vi "Dashboard custom_bartender&global&gripper&camera2.vi"() -> ()   [LabVIEW 2017]
uses:
  C:/Users/IMR Lab/Documents/LabVIEW Data/UniversalRobotsSDK_LABView/LabVIEW/Examples/LabVIEW10/UnderAutomation.UniversalRobots.dll
  UnderAutomation.UniversalRobots.dll
  Global 1.vi
panel:
  out "Rz부호":string
  out "Ry부호":string
  out "Rx부호":string
  out "RZ_havetogo":string
  out "RY_havetogo":string
  out "RX_havetogo":string
  out "Z_havetogo":string
  out "Y_havetogo":string
  out "X_havetogo":string
  out "지호씨가보낸 총좌표":string
  out "TCPOffsetRZ":dbl
  out "TCPOffsetRY":dbl
  out "TCPOffsetRX":dbl
  out "TCPOffsetZ":dbl
  out "TCPOffsetY":dbl
  out "TCPOffsetX":dbl
  out "3rd Order":bool
  out "2nd Order":bool
  out "1st Order":bool
  in  "stop":bool
  out "Rx":dbl
  out "Rz":dbl
  out "Ry":dbl
  out "Enabled":bool
  out "Port":i32
  in  "Move to particular posture":bool
  in  "Move to Zero position":bool
  out "Connected":bool
  in  "Robot IP(192.168.112.182)":string
  out "Connect error":errorcluster
  in  "Power on\nRelease brake":bool
  in  "Power off":bool
  in  "Connect":bool
  in  "Send script":bool
  in  "Script to execute":string
  out "Powered on":bool
  out "X":dbl
  out "Y":dbl
  out "Z":dbl
  out "License state":string
  # "랩뷰가 보여주는 RX RY RZ 는 신뢰x"
  # "movel(p[-0.0753945, -0.304532, 0.314608, -0.194623, 2.71667, -1.00228], a= 0.5, v=0.25)"
  # "movej( get_inverse_kin(p[0.3138, 0.0814, 0.1647, 0.4226, -2.3876, -2.3851]),  a=0.5, v=0.25, t=0, r=0)"
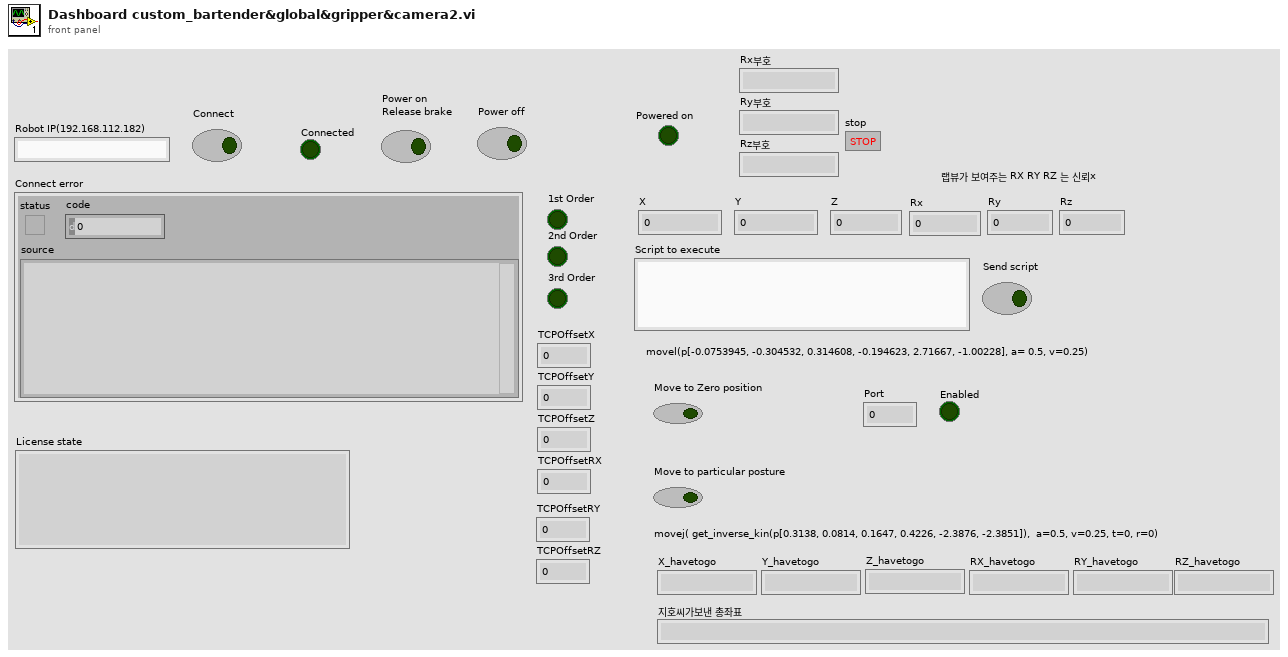
[diagram p1: front panel]
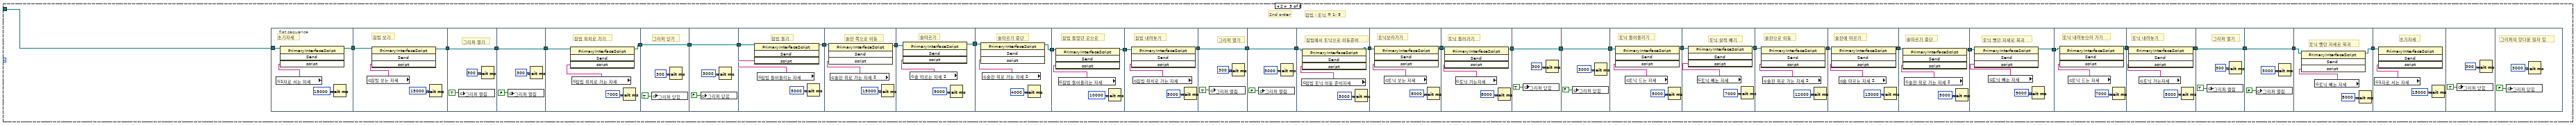
[diagram p14: hidden frame]
diagram:
  # "미니콜라 따르는 자세"
  # "술잔 중간지점 가는 자세"
  # "짐빔에서 토닉이동 준비 자세"
  # "술잔 따르는 자세2"
  # "술잔 위로 가는 자세2"
  # "토닉워터 뺴는 자세"
  # "토닉워 들어올리는 자세"
  # "토닉워터 가는 자세"
  # "토닉워터 보는 자세"
  # "짐빔 들어올리는 자세"
  # "짐빔로 가는 자세"
  # "짐빔 보는 자세"
  # "콜라 뺴는 자세"
  # "콜라 들어올리는 자세"
  # "콜라로 가는 자세"
  # "콜라 보는 자세"
  # "술잔 따르는 자세"
  # "술잔 위로 가는 자세"
  # "잭다니엘 들어올리는 자세"
  # "잭다니엘 위치로 가는 자세"
  # "잭다니엘 보는 자세"
  # "1자로 서는 자세"
  # "Example : Display power on status"
  # "Create a UR\ncobot instance"
  # "Show license state"
  # "Register your confidential license key to exit\ntrial period and use this library forever"
  # "Power off when button is clicked"
  # "Power on and release brake when button is clicked"
  # "Get your UR Dashboard interface"
  n1 = global write "Global 1.vi" "미니콜라 따르는 자세"("movej([-0.0902,-1.8120,-1.9241,-3.5769,6.2827,8.4658], a=0.5, v=0.25, t=0, r=0)") -> ()
  n2 = global write "Global 1.vi" "술잔 중간지점"("movej([-0.2173,-1.9485,-1.6874,-3.9352,6.2671,7.2276], a=0.5, v=0.25, t=0, r=0)") -> ()
  n3 = global write "Global 1.vi" "짐빔 토닉 이동 준비자세"("movej([-0.5421,-0.8131,0.8439,-0.0538,2.5052,5.9032], a=0.5, v=0.25, t=0, r=0)") -> ()
  n4 = global write "Global 1.vi" "잭다니엘 들어올리는 자세"("movej([0.8116,-2.0223,-1.2828,-3.0107,4.3284,5.9341], a=0.5, v=0.25, t=0, r=0)") -> ()
  n5 = global write "Global 1.vi" "잭다닐 위치로 가는 자세"("movej([0.8116,-2.3119,-1.606,-2.3958,4.3284,5.9341], a=0.5, v=0.25, t=0, r=0)") -> ()
  n6 = global write "Global 1.vi" "짐빔 들어올리는 자세"("movej([-0.5421,-0.8131,0.8439,-0.0538,2.5052,5.9032], a=0.5, v=0.25, t=0, r=0)") -> ()
  n7 = global write "Global 1.vi" "술잔 위로 가는 자세 2"("movej([0.0485,-1.6015,2.5780,-1.0382,-0.0520,5.3649], a=0.5, v=0.25, t=0, r=0)") -> ()
  n8 = global write "Global 1.vi" "1자로 서는 자세"("movej([3.1412,-1.5708,0,-1.5708,3.1412,5.8904], a=0.5, v=0.25, t=0, r=0)") -> ()
  n9 = global write "Global 1.vi" "짐빔 위치로 가는 자세"("movej([-0.5436,-0.4519,0.8428,-0.3534,2.6134,5.9032], a=0.5, v=0.25, t=0, r=0)") -> ()
  n10 = global write "Global 1.vi" "술잔 위로 가는 자세"("movej([-0.0903,-2.0548,-2.0169,-3.3289,6.2826,7.4091], a=0.5, v=0.25, t=0, r=0)") -> ()
  n11 = global write "Global 1.vi" "잭다니엘 보는 자세"("movej([0,-2.2170,-1.4226,-2.2842,3.1412,6.2832], a=0.5, v=0.25, t=0, r=0)") -> ()
  n12 = global write "Global 1.vi" "콜라 빼는 자세"("movej([0.8789,-1.5237,-2.1070,-2.6679, 3.9917,5.9085], a=0.5, v=0.25, t=0, r=0)") -> ()
  n13 = global write "Global 1.vi" "콜라 드는 자세"("movej([1.2020,-1.8452,-1.7403,-2.7082,4.3162,5.9158], a=0.5, v=0.25, t=0, r=0)") -> ()
  n14 = global write "Global 1.vi" "콜라 보는 자세"("movej([0,-1.8110,-2.1684,-2.3033,3.1543,5.9213], a=0.5, v=0.25, t=0, r=0)") -> ()
  n15 = global write "Global 1.vi" "콜라로 가는자세"("movej([1.2020,-2.166,-1.9385,-2.1863,4.3172,5.9210], a=0.5, v=0.25, t=0, r=0)") -> ()
  n16 = global write "Global 1.vi" "토닉 빼는 자세"("movej([-0.5277,-1.5104,1.5889,-0.0548,2.5728,5.9025], a=0.5, v=0.25, t=0, r=0)") -> ()
  n17 = global write "Global 1.vi" "술 따르는 자세 2"("movej([0.0412,-1.9708,2.4700,-1.0157,-0.0618,4.8998], a=0.5, v=0.25, t=0, r=0)") -> ()
  n18 = global write "Global 1.vi" "짐빔 보는 자세"("movej([-0.0364,-0.6154,0.9421,-0.3291,3.1047,5.9020], a=0.5, v=0.25, t=0, r=0)") -> ()
  n19 = global write "Global 1.vi" "토닉 드는 자세"("movej([-1.0311,-1.1460,1.5830,-0.4348,2.0708,5.9048], a=0.5, v=0.25, t=0, r=0)") -> ()
  n20 = global write "Global 1.vi" "토닉 보는 자세"("movej([-0.4690,-1.1292,2.1508,-1.0119,2.6124,5.9032], a=0.5, v=0.25, t=0, r=0)") -> ()
  n21 = global write "Global 1.vi" "술 따르는 자세"("movej([-0.0902,-1.9024,-1.9241,-3.5769,6.2827,8.4692], a=0.5, v=0.25, t=0, r=0)") -> ()
  n22 = global write "Global 1.vi" "토닉 가는자세"("movej([-0.9924,-0.8742,1.7459,-0.8837,2.0958,5.9048], a=0.5, v=0.25, t=0, r=0)") -> ()
  n23 = constructor class="UR"() -> (reference out=w25:refnum<k24>)  [unwired: 3 in, 2 out]
  n24 = while {
    tunnel: w25 -> [w31]
    stop <- FALSE stop-if-true
    # "Connect to the robot when button is pressed"
    # "Show if primary interface is connected"
    # "Get your UR primary interface"
    n25 = property class="UR"(reference=w31) -> ("PrimaryInterface"=w34:refnum<k24>)  [unwired: 1 in, 2 out]
    n26 = Wait (ms)(milliseconds to wait=u32 50) -> ()  [unwired: 1 out]
    n27 = property class="PrimaryInterfaceClientInternal"(reference=w34) -> ("Connected"=w33:bool)  [unwired: 1 in, 2 out]
    "Connected" <- w33
    n28 = case shown="True" "Connect" {
      tunnel: w31 -> [_ w478]
      frame False {
      }
      frame True {
        n29 = flat-sequence {
          tunnel: w478 -> [w480]
          frame #0 {
            n30 = invoke class="UR" method="Connect"(reference=w480, "ip"="Robot IP(192.168.112.182)") -> (error out=→"Connect error":errorcluster)  [unwired: 2 in, 3 out]
          }
        }
      }
    }
    n31 = case shown="True" w33 {
      tunnel: w34 -> [_ w40]
      frame False {
      }
      frame True {
        # "Send URScript when button pressed"
        # "Example : Display current cartesian pose"
        n32 = property class="PrimaryInterfaceClientInternal"(reference=w40) -> ("Script"=w48:refnum<k24>)  [unwired: 1 in, 2 out]
        n33 = global read "Global 1.vi" "2nd Order"() -> (w51:bool)
        "2nd Order" <- w51
        n34 = global read "Global 1.vi" "3rd Order"() -> (w50:bool)
        "3rd Order" <- w50
        n35 = global read "Global 1.vi" "1st Order"() -> (w52:bool)
        "1st Order" <- w52
        n36 = Build Array(w52, w51, w50) -> (w53:bool[])
        n37 = Boolean Array To Number(Boolean array=w53) -> (number=w49:u32)
        n38 = case shown="1" w49 {
          tunnel: w48 -> [_ w106 w313 _ _ _ _ _]
          frame 0, Default {
          }
          frame 1 {
            # "잭다 : 콜라 = 1 : 3"
            # "1st order"
            n39 = flat-sequence {
              tunnel: w106 -> [w110]
              tunnel: [w109] -> w105
              tunnel: w105 -> [w114]
              tunnel: [w112] -> w97
              tunnel: w97 -> [w117]
              tunnel: [w117] -> w95
              tunnel: w95 -> [w120]
              tunnel: [w120] -> w72
              tunnel: w72 -> [w124]
              tunnel: [w124] -> w69
              tunnel: w69 -> [w128]
              tunnel: [w128] -> w68
              tunnel: w68 -> [w190]
              tunnel: [w190] -> w71
              tunnel: w71 -> [w191]
              tunnel: [w191] -> w70
              tunnel: w70 -> [w195]
              tunnel: [w192] -> w96
              tunnel: w96 -> [w198]
              tunnel: [w198] -> w94
              tunnel: w94 -> [w201]
              tunnel: [w201] -> w93
              tunnel: w93 -> [w203]
              tunnel: [w202] -> w80
              tunnel: w80 -> [w207]
              tunnel: [w206] -> w79
              tunnel: w79 -> [w211]
              tunnel: [w210] -> w104
              tunnel: w104 -> [w216]
              tunnel: [w214] -> w103
              tunnel: w103 -> [w219]
              tunnel: [w218] -> w78
              tunnel: w78 -> [w223]
              tunnel: [w222] -> w77
              tunnel: [w226] -> w102
              tunnel: w77 -> [w228]
              tunnel: w102 -> [w231]
              tunnel: [w230] -> w92
              tunnel: w92 -> [w236]
              tunnel: [w236] -> w91
              tunnel: w91 -> [w239]
              tunnel: [w239] -> w90
              tunnel: w90 -> [w241]
              tunnel: [w240] -> w101
              tunnel: w101 -> [w245]
              tunnel: [w244] -> w89
              tunnel: w89 -> [w250]
              tunnel: [w250] -> w88
              tunnel: w88 -> [w253]
              tunnel: [w253] -> w87
              tunnel: w87 -> [w255]
              tunnel: [w254] -> w86
              tunnel: w86 -> [w259]
              tunnel: [w258] -> w76
              tunnel: w76 -> [w263]
              tunnel: [w262] -> w75
              tunnel: w75 -> [w267]
              tunnel: [w266] -> w100
              tunnel: w100 -> [w271]
              tunnel: [w270] -> w99
              tunnel: w99 -> [w275]
              tunnel: [w274] -> w74
              tunnel: w74 -> [w279]
              tunnel: [w278] -> w73
              tunnel: w73 -> [w283]
              tunnel: [w282] -> w85
              tunnel: w85 -> [w287]
              tunnel: [w286] -> w98
              tunnel: w98 -> [w291]
              tunnel: [w290] -> w83
              tunnel: [w294] -> w84
              tunnel: w83 -> [w294]
              tunnel: [w297] -> w82
              tunnel: w84 -> [w297]
              tunnel: w82 -> [w301]
              tunnel: [w300] -> w81
              tunnel: w81 -> [w304]
              frame #0 {
                # "초기자세"
                n40 = global read "Global 1.vi" "1자로 서는 자세"() -> (w108:string)
                n41 = invoke class="PrimaryInterfaceScript" method="Send"(reference=w110, "script"=w108) -> (reference out=w109:refnum<k24>)  [unwired: 2 in, 3 out]
                n42 = Wait (ms)(milliseconds to wait=u32 15000) -> ()  [unwired: 1 out]
              }
              frame #1 {
                # "잭다니엘 보기"
                n43 = global read "Global 1.vi" "잭다니엘 보는 자세"() -> (w113:string)
                n44 = invoke class="PrimaryInterfaceScript" method="Send"(reference=w114, "script"=w113) -> (reference out=w112:refnum<k24>)  [unwired: 2 in, 3 out]
                n45 = Wait (ms)(milliseconds to wait=u32 15000) -> ()  [unwired: 1 out]
              }
              frame #2 {
                # "그리퍼 열기"
                n46 = global write "Global 1.vi" "그리퍼 열림"(TRUE ("그리퍼 열림")) -> ()
                n47 = Wait (ms)(milliseconds to wait=u32 300) -> ()  [unwired: 1 out]
              }
              frame #3 {
                n48 = global write "Global 1.vi" "그리퍼 열림"(FALSE ("그리퍼 열림")) -> ()
                n49 = Wait (ms)(milliseconds to wait=u32 300) -> ()  [unwired: 1 out]
              }
              frame #4 {
                n50 = global write "Global 1.vi" "몇번 병을 볼것인가"("0" ("몇번 병을 볼것인가")) -> ()
                n51 = global write "Global 1.vi" "TCP 스위치"(TRUE ("그리퍼 열림")) -> ()
                n52 = Wait (ms)(milliseconds to wait=u32 300) -> ()  [unwired: 1 out]
              }
              frame #5 {
                n53 = local read "Rx부호"() -> (w127:string)
                n54 = local read "Ry부호"() -> (w126:string)
                n55 = local read "Rz부호"() -> (w125:string)
                n56 = case shown="\"1\"" w125 {
                  frame "False", Default {
                  }
                  frame "True" {
                  }
                  frame "2" {
                  }
                  frame "1" {
                    n57 = local read "RZ_havetogo"() -> (w133:string)
                    n58 = Decimal String To Number(string=w133) -> (number=w132:i32)  [unwired: 2 in, 1 out]
                    n59 = To Double Precision Float(number=w132) -> (double precision float=w131:dbl)
                    n60 = Format Into String(format string="-%f", w131) -> (resulting string=w129:string)  [unwired: 2 in, 1 out]
                    n61 = local write "RZ_havetogo"(w129) -> ()
                  }
                }
                n62 = case shown="\"1\"" w126 {
                  frame "False", Default {
                  }
                  frame "True" {
                  }
                  frame "2" {
                  }
                  frame "1" {
                    n63 = local read "RY_havetogo"() -> (w138:string)
                    n64 = Decimal String To Number(string=w138) -> (number=w137:i32)  [unwired: 2 in, 1 out]
                    n65 = To Double Precision Float(number=w137) -> (double precision float=w134:dbl)
                    n66 = Format Into String(format string="-%f", w134) -> (resulting string=w135:string)  [unwired: 2 in, 1 out]
                    n67 = local write "RY_havetogo"(w135) -> ()
                  }
                }
                n68 = case shown="\"1\"" w127 {
                  frame "False", Default {
                  }
                  frame "True" {
                  }
                  frame "2" {
                  }
                  frame "1" {
                    n69 = local read "RX_havetogo"() -> (w143:string)
                    n70 = Decimal String To Number(string=w143) -> (number=w142:i32)  [unwired: 2 in, 1 out]
                    n71 = To Double Precision Float(number=w142) -> (double precision float=w141:dbl)
                    n72 = Format Into String(format string="-%f", w141) -> (resulting string=w139:string)  [unwired: 2 in, 1 out]
                    n73 = local write "RX_havetogo"(w139) -> ()
                  }
                }
              }
              frame #6 {
                n74 = local read "RZ_havetogo"() -> (w182:string)
                n75 = local read "RY_havetogo"() -> (w183:string)
                n76 = local read "Y_havetogo"() -> (w186:string)
                n77 = local read "Z_havetogo"() -> (w185:string)
                n78 = local read "RX_havetogo"() -> (w184:string)
                n79 = local read "X_havetogo"() -> (w187:string)
                n80 = Decimal String To Number(string=w185) -> (number=w173:i32)  [unwired: 2 in, 1 out]
                n81 = Decimal String To Number(string=w187) -> (number=w179:i32)  [unwired: 2 in, 1 out]
                n82 = Decimal String To Number(string=w186) -> (number=w176:i32)  [unwired: 2 in, 1 out]
                n83 = Decimal String To Number(string=w184) -> (number=w170:i32)  [unwired: 2 in, 1 out]
                n84 = Decimal String To Number(string=w183) -> (number=w167:i32)  [unwired: 2 in, 1 out]
                n85 = Decimal String To Number(string=w182) -> (number=w164:i32)  [unwired: 2 in, 1 out]
                n86 = To Double Precision Float(number=w179) -> (double precision float=w181:dbl)
                n87 = To Double Precision Float(number=w173) -> (double precision float=w175:dbl)
                n88 = To Double Precision Float(number=w176) -> (double precision float=w178:dbl)
                n89 = To Double Precision Float(number=w170) -> (double precision float=w172:dbl)
                n90 = To Double Precision Float(number=w167) -> (double precision float=w169:dbl)
                n91 = local read "X"() -> (w151:dbl)
                n92 = Multiply(x=w181, y=0.001) -> (x*y=w163:dbl)
                n93 = Multiply(x=w175, y=0.001) -> (x*y=w159:dbl)
                n94 = Multiply(x=w178, y=0.001) -> (x*y=w161:dbl)
                n95 = Multiply(x=w172, y=0.001) -> (x*y=w157:dbl)
                n96 = Multiply(x=w169, y=0.001) -> (x*y=w155:dbl)
                n97 = local read "Y"() -> (w150:dbl)
                n98 = local read "Z"() -> (w149:dbl)
                n99 = To Double Precision Float(number=w164) -> (double precision float=w166:dbl)
                n100 = Add(x=w151, y=w163) -> (x+y=w162:dbl)
                n101 = local read "Rx"() -> (w148:dbl)
                n102 = Multiply(x=w166, y=0.001) -> (x*y=w153:dbl)
                n103 = Add(x=w159, y=w149) -> (x+y=w158:dbl)
                n104 = Add(x=w161, y=w150) -> (x+y=w160:dbl)
                n105 = local read "Ry"() -> (w147:dbl)
                n106 = local read "Rz"() -> (w146:dbl)
                n107 = Add(x=w157, y=w148) -> (x+y=w156:dbl)
                n108 = Add(x=w155, y=w147) -> (x+y=w154:dbl)
                n109 = Add(x=w153, y=w146) -> (x+y=w152:dbl)
                n110 = Format Into String(format string="movej( get_inverse_kin(p[%f, %f, %f, %f, %f, %f]), a= 0.5, v=0.25, t=0, r=0)", w162, w160, w158, w156, w154, w152) -> (resulting string=w144:string)  [unwired: 2 in, 1 out]
                n111 = global write "Global 1.vi" "잭다닐 위치로 가는 자세"(w144) -> ()
                n112 = global write "Global 1.vi" "TCP 스위치"(FALSE ("그리퍼 열림")) -> ()
                n113 = Wait (ms)(milliseconds to wait=u32 300) -> ()  [unwired: 1 out]
              }
              frame #7 {
              }
              frame #8 {
                # "잭다니엘 위치로 가기"
                n114 = global read "Global 1.vi" "잭다닐 위치로 가는 자세"() -> (w194:string)
                n115 = invoke class="PrimaryInterfaceScript" method="Send"(reference=w195, "script"=w194) -> (reference out=w192:refnum<k24>)  [unwired: 2 in, 3 out]
                n116 = Wait (ms)(milliseconds to wait=u32 7000) -> ()  [unwired: 1 out]
              }
              frame #9 {
                # "그리퍼 닫기"
                n117 = global write "Global 1.vi" "그리퍼 닫힘"(TRUE ("그리퍼 열림")) -> ()
                n118 = Wait (ms)(milliseconds to wait=u32 300) -> ()  [unwired: 1 out]
              }
              frame #10 {
                n119 = global write "Global 1.vi" "그리퍼 닫힘"(FALSE ("그리퍼 열림")) -> ()
                n120 = Wait (ms)(milliseconds to wait=u32 3000) -> ()  [unwired: 1 out]
              }
              frame #11 {
                # "잭다니엘 들기"
                n121 = global read "Global 1.vi" "잭다니엘 들어올리는 자세"() -> (w205:string)
                n122 = invoke class="PrimaryInterfaceScript" method="Send"(reference=w203, "script"=w205) -> (reference out=w202:refnum<k24>)  [unwired: 2 in, 3 out]
                n123 = Wait (ms)(milliseconds to wait=u32 3000) -> ()  [unwired: 1 out]
              }
              frame #12 {
                # "술잔 중간지점으로 이동"
                n124 = global read "Global 1.vi" "술잔 중간지점"() -> (w208:string)
                n125 = invoke class="PrimaryInterfaceScript" method="Send"(reference=w207, "script"=w208) -> (reference out=w206:refnum<k24>)  [unwired: 2 in, 3 out]
                n126 = Wait (ms)(milliseconds to wait=u32 15000) -> ()  [unwired: 1 out]
              }
              frame #13 {
                # "술잔 쪽으로 이동"
                n127 = global read "Global 1.vi" "술잔 위로 가는 자세"() -> (w212:string)
                n128 = invoke class="PrimaryInterfaceScript" method="Send"(reference=w211, "script"=w212) -> (reference out=w210:refnum<k24>)  [unwired: 2 in, 3 out]
                n129 = Wait (ms)(milliseconds to wait=u32 5000) -> ()  [unwired: 1 out]
              }
              frame #14 {
                # "술따르기"
                n130 = global read "Global 1.vi" "술 따르는 자세"() -> (w215:string)
                n131 = invoke class="PrimaryInterfaceScript" method="Send"(reference=w216, "script"=w215) -> (reference out=w214:refnum<k24>)  [unwired: 2 in, 3 out]
                n132 = Wait (ms)(milliseconds to wait=u32 9000) -> ()  [unwired: 1 out]
              }
              frame #15 {
                # "술따르기 중단"
                n133 = global read "Global 1.vi" "술잔 위로 가는 자세"() -> (w220:string)
                n134 = invoke class="PrimaryInterfaceScript" method="Send"(reference=w219, "script"=w220) -> (reference out=w218:refnum<k24>)  [unwired: 2 in, 3 out]
                n135 = Wait (ms)(milliseconds to wait=u32 4000) -> ()  [unwired: 1 out]
              }
              frame #16 {
                # "술잔 중간지점으로 이동"
                n136 = global read "Global 1.vi" "술잔 중간지점"() -> (w224:string)
                n137 = invoke class="PrimaryInterfaceScript" method="Send"(reference=w223, "script"=w224) -> (reference out=w222:refnum<k24>)  [unwired: 2 in, 3 out]
                n138 = Wait (ms)(milliseconds to wait=u32 7000) -> ()  [unwired: 1 out]
              }
              frame #17 {
                # "잭다니엘 들었던 곳으로"
                n139 = global read "Global 1.vi" "잭다니엘 들어올리는 자세"() -> (w227:string)
                n140 = invoke class="PrimaryInterfaceScript" method="Send"(reference=w228, "script"=w227) -> (reference out=w226:refnum<k24>)  [unwired: 2 in, 3 out]
                n141 = Wait (ms)(milliseconds to wait=u32 10000) -> ()  [unwired: 1 out]
              }
              frame #18 {
                # "잭다니엘 내려놓기"
                n142 = global read "Global 1.vi" "잭다닐 위치로 가는 자세"() -> (w233:string)
                n143 = invoke class="PrimaryInterfaceScript" method="Send"(reference=w231, "script"=w233) -> (reference out=w230:refnum<k24>)  [unwired: 2 in, 3 out]
                n144 = Wait (ms)(milliseconds to wait=u32 5000) -> ()  [unwired: 1 out]
              }
              frame #19 {
                # "그리퍼 열기"
                n145 = global write "Global 1.vi" "그리퍼 열림"(TRUE ("그리퍼 열림")) -> ()
                n146 = Wait (ms)(milliseconds to wait=u32 300) -> ()  [unwired: 1 out]
              }
              frame #20 {
                n147 = global write "Global 1.vi" "그리퍼 열림"(FALSE ("그리퍼 열림")) -> ()
                n148 = Wait (ms)(milliseconds to wait=u32 3000) -> ()  [unwired: 1 out]
              }
              frame #21 {
                # "콜라보러가기"
                n149 = global read "Global 1.vi" "콜라 보는 자세"() -> (w243:string)
                n150 = invoke class="PrimaryInterfaceScript" method="Send"(reference=w241, "script"=w243) -> (reference out=w240:refnum<k24>)  [unwired: 2 in, 3 out]
                n151 = Wait (ms)(milliseconds to wait=u32 8000) -> ()  [unwired: 1 out]
              }
              frame #22 {
                # "콜라 들러가기"
                n152 = global read "Global 1.vi" "콜라로 가는자세"() -> (w247:string)
                n153 = invoke class="PrimaryInterfaceScript" method="Send"(reference=w245, "script"=w247) -> (reference out=w244:refnum<k24>)  [unwired: 2 in, 3 out]
                n154 = Wait (ms)(milliseconds to wait=u32 8000) -> ()  [unwired: 1 out]
              }
              frame #23 {
                n155 = global write "Global 1.vi" "그리퍼 닫힘"(TRUE ("그리퍼 열림")) -> ()
                n156 = Wait (ms)(milliseconds to wait=u32 300) -> ()  [unwired: 1 out]
              }
              frame #24 {
                n157 = global write "Global 1.vi" "그리퍼 닫힘"(FALSE ("그리퍼 열림")) -> ()
                n158 = Wait (ms)(milliseconds to wait=u32 3000) -> ()  [unwired: 1 out]
              }
              frame #25 {
                # "콜라 들어올리기"
                n159 = global read "Global 1.vi" "콜라 드는 자세"() -> (w257:string)
                n160 = invoke class="PrimaryInterfaceScript" method="Send"(reference=w255, "script"=w257) -> (reference out=w254:refnum<k24>)  [unwired: 2 in, 3 out]
                n161 = Wait (ms)(milliseconds to wait=u32 5000) -> ()  [unwired: 1 out]
              }
              frame #26 {
                # "콜라 살짝 빼기"
                n162 = global read "Global 1.vi" "콜라 빼는 자세"() -> (w261:string)
                n163 = invoke class="PrimaryInterfaceScript" method="Send"(reference=w259, "script"=w261) -> (reference out=w258:refnum<k24>)  [unwired: 2 in, 3 out]
                n164 = Wait (ms)(milliseconds to wait=u32 5000) -> ()  [unwired: 1 out]
              }
              frame #27 {
                # "술잔 중간지점으로 이동"
                n165 = global read "Global 1.vi" "술잔 중간지점"() -> (w264:string)
                n166 = invoke class="PrimaryInterfaceScript" method="Send"(reference=w263, "script"=w264) -> (reference out=w262:refnum<k24>)  [unwired: 2 in, 3 out]
                n167 = Wait (ms)(milliseconds to wait=u32 15000) -> ()  [unwired: 1 out]
              }
              frame #28 {
                # "술잔으로 이동"
                n168 = global read "Global 1.vi" "술잔 위로 가는 자세"() -> (w269:string)
                n169 = invoke class="PrimaryInterfaceScript" method="Send"(reference=w267, "script"=w269) -> (reference out=w266:refnum<k24>)  [unwired: 2 in, 3 out]
                n170 = Wait (ms)(milliseconds to wait=u32 5000) -> ()  [unwired: 1 out]
              }
              frame #29 {
                # "미니콜라에 따르기"
                n171 = global read "Global 1.vi" "미니콜라 따르는 자세"() -> (w273:string)
                n172 = invoke class="PrimaryInterfaceScript" method="Send"(reference=w271, "script"=w273) -> (reference out=w270:refnum<k24>)  [unwired: 2 in, 3 out]
                n173 = Wait (ms)(milliseconds to wait=u32 11000) -> ()  [unwired: 1 out]
              }
              frame #30 {
                # "술따르기 중단"
                n174 = global read "Global 1.vi" "술잔 위로 가는 자세"() -> (w277:string)
                n175 = invoke class="PrimaryInterfaceScript" method="Send"(reference=w275, "script"=w277) -> (reference out=w274:refnum<k24>)  [unwired: 2 in, 3 out]
                n176 = Wait (ms)(milliseconds to wait=u32 5000) -> ()  [unwired: 1 out]
              }
              frame #31 {
                # "술잔 중간지점으로 이동"
                n177 = global read "Global 1.vi" "술잔 중간지점"() -> (w280:string)
                n178 = invoke class="PrimaryInterfaceScript" method="Send"(reference=w279, "script"=w280) -> (reference out=w278:refnum<k24>)  [unwired: 2 in, 3 out]
                n179 = Wait (ms)(milliseconds to wait=u32 7000) -> ()  [unwired: 1 out]
              }
              frame #32 {
                # "콜라 뻇던 자세로 복귀"
                n180 = global read "Global 1.vi" "콜라 빼는 자세"() -> (w284:string)
                n181 = invoke class="PrimaryInterfaceScript" method="Send"(reference=w283, "script"=w284) -> (reference out=w282:refnum<k24>)  [unwired: 2 in, 3 out]
                n182 = Wait (ms)(milliseconds to wait=u32 7000) -> ()  [unwired: 1 out]
              }
              frame #33 {
                # "콜라 내려놓으러 가기"
                n183 = global read "Global 1.vi" "콜라 드는 자세"() -> (w289:string)
                n184 = invoke class="PrimaryInterfaceScript" method="Send"(reference=w287, "script"=w289) -> (reference out=w286:refnum<k24>)  [unwired: 2 in, 3 out]
                n185 = Wait (ms)(milliseconds to wait=u32 10000) -> ()  [unwired: 1 out]
              }
              frame #34 {
                # "콜라 내려놓기"
                n186 = global read "Global 1.vi" "콜라로 가는자세"() -> (w293:string)
                n187 = invoke class="PrimaryInterfaceScript" method="Send"(reference=w291, "script"=w293) -> (reference out=w290:refnum<k24>)  [unwired: 2 in, 3 out]
                n188 = Wait (ms)(milliseconds to wait=u32 5000) -> ()  [unwired: 1 out]
              }
              frame #35 {
                # "그리퍼 열기"
                n189 = global write "Global 1.vi" "그리퍼 열림"(TRUE ("그리퍼 열림")) -> ()
                n190 = Wait (ms)(milliseconds to wait=u32 300) -> ()  [unwired: 1 out]
              }
              frame #36 {
                n191 = global write "Global 1.vi" "그리퍼 열림"(FALSE ("그리퍼 열림")) -> ()
                n192 = Wait (ms)(milliseconds to wait=u32 3000) -> ()  [unwired: 1 out]
              }
              frame #37 {
                # "콜라 뻇던 자세로 복귀"
                n193 = global read "Global 1.vi" "콜라 빼는 자세"() -> (w302:string)
                n194 = invoke class="PrimaryInterfaceScript" method="Send"(reference=w301, "script"=w302) -> (reference out=w300:refnum<k24>)  [unwired: 2 in, 3 out]
                n195 = Wait (ms)(milliseconds to wait=u32 5000) -> ()  [unwired: 1 out]
              }
              frame #38 {
                # "초기자세"
                n196 = global read "Global 1.vi" "1자로 서는 자세"() -> (w306:string)
                n197 = invoke class="PrimaryInterfaceScript" method="Send"(reference=w304, "script"=w306) -> ()  [unwired: 2 in, 4 out]
                n198 = Wait (ms)(milliseconds to wait=u32 15000) -> ()  [unwired: 1 out]
              }
              frame #39 {
                n199 = global write "Global 1.vi" "그리퍼 닫힘"(TRUE ("그리퍼 열림")) -> ()
                n200 = Wait (ms)(milliseconds to wait=u32 300) -> ()  [unwired: 1 out]
              }
              frame #40 {
                # "그리퍼의 앙다문 일자 입"
                n201 = global write "Global 1.vi" "그리퍼 닫힘"(FALSE ("그리퍼 열림")) -> ()
                n202 = Wait (ms)(milliseconds to wait=u32 3000) -> ()  [unwired: 1 out]
              }
            }
          }
          frame 2 {
            # "짐빔 : 토닉 = 1: 3"
            # "2nd order"
            n203 = flat-sequence {
              tunnel: w313 -> [w346]
              tunnel: [w345] -> w342
              tunnel: w342 -> [w350]
              tunnel: [w348] -> w341
              tunnel: w341 -> [w353]
              tunnel: [w353] -> w340
              tunnel: w340 -> [w356]
              tunnel: [w356] -> w339
              tunnel: w339 -> [w360]
              tunnel: [w357] -> w338
              tunnel: w338 -> [w363]
              tunnel: [w363] -> w337
              tunnel: w337 -> [w366]
              tunnel: [w366] -> w336
              tunnel: w336 -> [w368]
              tunnel: [w367] -> w335
              tunnel: w335 -> [w372]
              tunnel: [w371] -> w334
              tunnel: w334 -> [w377]
              tunnel: [w375] -> w333
              tunnel: w333 -> [w380]
              tunnel: [w379] -> w332
              tunnel: w332 -> [w385]
              tunnel: [w383] -> w331
              tunnel: w331 -> [w388]
              tunnel: [w387] -> w330
              tunnel: w330 -> [w393]
              tunnel: [w393] -> w329
              tunnel: w329 -> [w396]
              tunnel: [w396] -> w312
              tunnel: w312 -> [w398]
              tunnel: [w397] -> w311
              tunnel: [w401] -> w328
              tunnel: w311 -> [w402]
              tunnel: w328 -> [w406]
              tunnel: [w405] -> w327
              tunnel: w327 -> [w411]
              tunnel: [w411] -> w326
              tunnel: w326 -> [w414]
              tunnel: [w414] -> w325
              tunnel: w325 -> [w416]
              tunnel: [w415] -> w324
              tunnel: w324 -> [w420]
              tunnel: [w419] -> w323
              tunnel: w323 -> [w424]
              tunnel: [w423] -> w322
              tunnel: w322 -> [w428]
              tunnel: [w427] -> w321
              tunnel: w321 -> [w432]
              tunnel: [w431] -> w320
              tunnel: w320 -> [w436]
              tunnel: [w435] -> w319
              tunnel: w319 -> [w440]
              tunnel: [w439] -> w318
              tunnel: w318 -> [w444]
              tunnel: [w443] -> w317
              tunnel: [w447] -> w316
              tunnel: w317 -> [w447]
              tunnel: [w450] -> w315
              tunnel: w316 -> [w450]
              tunnel: w315 -> [w454]
              tunnel: [w453] -> w314
              tunnel: w314 -> [w457]
              frame #0 {
                # "초기자세"
                n204 = global read "Global 1.vi" "1자로 서는 자세"() -> (w344:string)
                n205 = invoke class="PrimaryInterfaceScript" method="Send"(reference=w346, "script"=w344) -> (reference out=w345:refnum<k24>)  [unwired: 2 in, 3 out]
                n206 = Wait (ms)(milliseconds to wait=u32 15000) -> ()  [unwired: 1 out]
              }
              frame #1 {
                # "짐빔 보기"
                n207 = global read "Global 1.vi" "짐빔 보는 자세"() -> (w349:string)
                n208 = invoke class="PrimaryInterfaceScript" method="Send"(reference=w350, "script"=w349) -> (reference out=w348:refnum<k24>)  [unwired: 2 in, 3 out]
                n209 = Wait (ms)(milliseconds to wait=u32 15000) -> ()  [unwired: 1 out]
              }
              frame #2 {
                # "그리퍼 열기"
                n210 = global write "Global 1.vi" "그리퍼 열림"(TRUE ("그리퍼 열림")) -> ()
                n211 = Wait (ms)(milliseconds to wait=u32 300) -> ()  [unwired: 1 out]
              }
              frame #3 {
                n212 = global write "Global 1.vi" "그리퍼 열림"(FALSE ("그리퍼 열림")) -> ()
                n213 = Wait (ms)(milliseconds to wait=u32 300) -> ()  [unwired: 1 out]
              }
              frame #4 {
                # "짐빔 위치로 가기"
                n214 = global read "Global 1.vi" "짐빔 위치로 가는 자세"() -> (w359:string)
                n215 = invoke class="PrimaryInterfaceScript" method="Send"(reference=w360, "script"=w359) -> (reference out=w357:refnum<k24>)  [unwired: 2 in, 3 out]
                n216 = Wait (ms)(milliseconds to wait=u32 7000) -> ()  [unwired: 1 out]
              }
              frame #5 {
                # "그리퍼 닫기"
                n217 = global write "Global 1.vi" "그리퍼 닫힘"(TRUE ("그리퍼 열림")) -> ()
                n218 = Wait (ms)(milliseconds to wait=u32 300) -> ()  [unwired: 1 out]
              }
              frame #6 {
                n219 = global write "Global 1.vi" "그리퍼 닫힘"(FALSE ("그리퍼 열림")) -> ()
                n220 = Wait (ms)(milliseconds to wait=u32 3000) -> ()  [unwired: 1 out]
              }
              frame #7 {
                # "짐빔 들기"
                n221 = global read "Global 1.vi" "짐빔 들어올리는 자세"() -> (w370:string)
                n222 = invoke class="PrimaryInterfaceScript" method="Send"(reference=w368, "script"=w370) -> (reference out=w367:refnum<k24>)  [unwired: 2 in, 3 out]
                n223 = Wait (ms)(milliseconds to wait=u32 5000) -> ()  [unwired: 1 out]
              }
              frame #8 {
                # "술잔 쪽으로 이동"
                n224 = global read "Global 1.vi" "술잔 위로 가는 자세 2"() -> (w373:string)
                n225 = invoke class="PrimaryInterfaceScript" method="Send"(reference=w372, "script"=w373) -> (reference out=w371:refnum<k24>)  [unwired: 2 in, 3 out]
                n226 = Wait (ms)(milliseconds to wait=u32 15000) -> ()  [unwired: 1 out]
              }
              frame #9 {
                # "술따르기"
                n227 = global read "Global 1.vi" "술 따르는 자세 2"() -> (w376:string)
                n228 = invoke class="PrimaryInterfaceScript" method="Send"(reference=w377, "script"=w376) -> (reference out=w375:refnum<k24>)  [unwired: 2 in, 3 out]
                n229 = Wait (ms)(milliseconds to wait=u32 9000) -> ()  [unwired: 1 out]
              }
              frame #10 {
                # "술따르기 중단"
                n230 = global read "Global 1.vi" "술잔 위로 가는 자세 2"() -> (w381:string)
                n231 = invoke class="PrimaryInterfaceScript" method="Send"(reference=w380, "script"=w381) -> (reference out=w379:refnum<k24>)  [unwired: 2 in, 3 out]
                n232 = Wait (ms)(milliseconds to wait=u32 4000) -> ()  [unwired: 1 out]
              }
              frame #11 {
                # "짐빔 들었던 곳으로"
                n233 = global read "Global 1.vi" "짐빔 들어올리는 자세"() -> (w384:string)
                n234 = invoke class="PrimaryInterfaceScript" method="Send"(reference=w385, "script"=w384) -> (reference out=w383:refnum<k24>)  [unwired: 2 in, 3 out]
                n235 = Wait (ms)(milliseconds to wait=u32 10000) -> ()  [unwired: 1 out]
              }
              frame #12 {
                # "짐빔 내려놓기"
                n236 = global read "Global 1.vi" "짐빔 위치로 가는 자세"() -> (w390:string)
                n237 = invoke class="PrimaryInterfaceScript" method="Send"(reference=w388, "script"=w390) -> (reference out=w387:refnum<k24>)  [unwired: 2 in, 3 out]
                n238 = Wait (ms)(milliseconds to wait=u32 5000) -> ()  [unwired: 1 out]
              }
              frame #13 {
                # "그리퍼 열기"
                n239 = global write "Global 1.vi" "그리퍼 열림"(TRUE ("그리퍼 열림")) -> ()
                n240 = Wait (ms)(milliseconds to wait=u32 300) -> ()  [unwired: 1 out]
              }
              frame #14 {
                n241 = global write "Global 1.vi" "그리퍼 열림"(FALSE ("그리퍼 열림")) -> ()
                n242 = Wait (ms)(milliseconds to wait=u32 3000) -> ()  [unwired: 1 out]
              }
              frame #15 {
                # "짐빔에서 토닉으로 이동준비"
                n243 = global read "Global 1.vi" "짐빔 토닉 이동 준비자세"() -> (w400:string)
                n244 = invoke class="PrimaryInterfaceScript" method="Send"(reference=w398, "script"=w400) -> (reference out=w397:refnum<k24>)  [unwired: 2 in, 3 out]
                n245 = Wait (ms)(milliseconds to wait=u32 5000) -> ()  [unwired: 1 out]
              }
              frame #16 {
                # "토닉보러가기"
                n246 = global read "Global 1.vi" "토닉 보는 자세"() -> (w404:string)
                n247 = invoke class="PrimaryInterfaceScript" method="Send"(reference=w402, "script"=w404) -> (reference out=w401:refnum<k24>)  [unwired: 2 in, 3 out]
                n248 = Wait (ms)(milliseconds to wait=u32 8000) -> ()  [unwired: 1 out]
              }
              frame #17 {
                # "토닉 들러가기"
                n249 = global read "Global 1.vi" "토닉 가는자세"() -> (w408:string)
                n250 = invoke class="PrimaryInterfaceScript" method="Send"(reference=w406, "script"=w408) -> (reference out=w405:refnum<k24>)  [unwired: 2 in, 3 out]
                n251 = Wait (ms)(milliseconds to wait=u32 8000) -> ()  [unwired: 1 out]
              }
              frame #18 {
                n252 = global write "Global 1.vi" "그리퍼 닫힘"(TRUE ("그리퍼 열림")) -> ()
                n253 = Wait (ms)(milliseconds to wait=u32 300) -> ()  [unwired: 1 out]
              }
              frame #19 {
                n254 = global write "Global 1.vi" "그리퍼 닫힘"(FALSE ("그리퍼 열림")) -> ()
                n255 = Wait (ms)(milliseconds to wait=u32 3000) -> ()  [unwired: 1 out]
              }
              frame #20 {
                # "토닉 들어올리기"
                n256 = global read "Global 1.vi" "토닉 드는 자세"() -> (w418:string)
                n257 = invoke class="PrimaryInterfaceScript" method="Send"(reference=w416, "script"=w418) -> (reference out=w415:refnum<k24>)  [unwired: 2 in, 3 out]
                n258 = Wait (ms)(milliseconds to wait=u32 5000) -> ()  [unwired: 1 out]
              }
              frame #21 {
                # "토닉 살짝 빼기"
                n259 = global read "Global 1.vi" "토닉 빼는 자세"() -> (w422:string)
                n260 = invoke class="PrimaryInterfaceScript" method="Send"(reference=w420, "script"=w422) -> (reference out=w419:refnum<k24>)  [unwired: 2 in, 3 out]
                n261 = Wait (ms)(milliseconds to wait=u32 7000) -> ()  [unwired: 1 out]
              }
              frame #22 {
                # "술잔으로 이동"
                n262 = global read "Global 1.vi" "술잔 위로 가는 자세 2"() -> (w426:string)
                n263 = invoke class="PrimaryInterfaceScript" method="Send"(reference=w424, "script"=w426) -> (reference out=w423:refnum<k24>)  [unwired: 2 in, 3 out]
                n264 = Wait (ms)(milliseconds to wait=u32 12000) -> ()  [unwired: 1 out]
              }
              frame #23 {
                # "술잔에 따르기"
                n265 = global read "Global 1.vi" "술 따르는 자세 2"() -> (w430:string)
                n266 = invoke class="PrimaryInterfaceScript" method="Send"(reference=w428, "script"=w430) -> (reference out=w427:refnum<k24>)  [unwired: 2 in, 3 out]
                n267 = Wait (ms)(milliseconds to wait=u32 13000) -> ()  [unwired: 1 out]
              }
              frame #24 {
                # "술따르기 중단"
                n268 = global read "Global 1.vi" "술잔 위로 가는 자세 2"() -> (w434:string)
                n269 = invoke class="PrimaryInterfaceScript" method="Send"(reference=w432, "script"=w434) -> (reference out=w431:refnum<k24>)  [unwired: 2 in, 3 out]
                n270 = Wait (ms)(milliseconds to wait=u32 5000) -> ()  [unwired: 1 out]
              }
              frame #25 {
                # "토닉 뻇던 자세로 복귀"
                n271 = global read "Global 1.vi" "토닉 빼는 자세"() -> (w437:string)
                n272 = invoke class="PrimaryInterfaceScript" method="Send"(reference=w436, "script"=w437) -> (reference out=w435:refnum<k24>)  [unwired: 2 in, 3 out]
                n273 = Wait (ms)(milliseconds to wait=u32 9000) -> ()  [unwired: 1 out]
              }
              frame #26 {
                # "토닉 내려놓으러 가기"
                n274 = global read "Global 1.vi" "토닉 드는 자세"() -> (w442:string)
                n275 = invoke class="PrimaryInterfaceScript" method="Send"(reference=w440, "script"=w442) -> (reference out=w439:refnum<k24>)  [unwired: 2 in, 3 out]
                n276 = Wait (ms)(milliseconds to wait=u32 7000) -> ()  [unwired: 1 out]
              }
              frame #27 {
                # "토닉 내려놓기"
                n277 = global read "Global 1.vi" "토닉 가는자세"() -> (w446:string)
                n278 = invoke class="PrimaryInterfaceScript" method="Send"(reference=w444, "script"=w446) -> (reference out=w443:refnum<k24>)  [unwired: 2 in, 3 out]
                n279 = Wait (ms)(milliseconds to wait=u32 5000) -> ()  [unwired: 1 out]
              }
              frame #28 {
                # "그리퍼 열기"
                n280 = global write "Global 1.vi" "그리퍼 열림"(TRUE ("그리퍼 열림")) -> ()
                n281 = Wait (ms)(milliseconds to wait=u32 300) -> ()  [unwired: 1 out]
              }
              frame #29 {
                n282 = global write "Global 1.vi" "그리퍼 열림"(FALSE ("그리퍼 열림")) -> ()
                n283 = Wait (ms)(milliseconds to wait=u32 3000) -> ()  [unwired: 1 out]
              }
              frame #30 {
                # "토닉 뻇던 자세로 복귀"
                n284 = global read "Global 1.vi" "토닉 빼는 자세"() -> (w455:string)
                n285 = invoke class="PrimaryInterfaceScript" method="Send"(reference=w454, "script"=w455) -> (reference out=w453:refnum<k24>)  [unwired: 2 in, 3 out]
                n286 = Wait (ms)(milliseconds to wait=u32 5000) -> ()  [unwired: 1 out]
              }
              frame #31 {
                # "초기자세"
                n287 = global read "Global 1.vi" "1자로 서는 자세"() -> (w459:string)
                n288 = invoke class="PrimaryInterfaceScript" method="Send"(reference=w457, "script"=w459) -> ()  [unwired: 2 in, 4 out]
                n289 = Wait (ms)(milliseconds to wait=u32 15000) -> ()  [unwired: 1 out]
              }
              frame #32 {
                n290 = global write "Global 1.vi" "그리퍼 닫힘"(TRUE ("그리퍼 열림")) -> ()
                n291 = Wait (ms)(milliseconds to wait=u32 300) -> ()  [unwired: 1 out]
              }
              frame #33 {
                # "그리퍼의 앙다문 일자 입"
                n292 = global write "Global 1.vi" "그리퍼 닫힘"(FALSE ("그리퍼 열림")) -> ()
                n293 = Wait (ms)(milliseconds to wait=u32 3000) -> ()  [unwired: 1 out]
              }
            }
          }
          frame 3 {
            # "multi order"
          }
          frame 4 {
            # "짐빔 : 우유 = 1 : 3"
            # "3rd order"
          }
          frame 5 {
            # "multi order"
          }
          frame 6 {
            # "multi order"
          }
          frame 7 {
            # "multi order"
          }
        }
        n294 = case shown="True" "Send script" {
          tunnel: w48 -> [_ w470]
          frame False {
          }
          frame True {
            n295 = flat-sequence {
              tunnel: w470 -> [w472]
              frame #0 {
                n296 = invoke class="PrimaryInterfaceScript" method="Send"(reference=w472, "script"="Script to execute") -> ()  [unwired: 2 in, 4 out]
              }
            }
          }
        }
        n297 = case shown="True" "Move to Zero position" {
          tunnel: w48 -> [_ w467]
          frame False {
          }
          frame True {
            n298 = flat-sequence {
              tunnel: w467 -> [w469]
              frame #0 {
                n299 = invoke class="PrimaryInterfaceScript" method="Send"(reference=w469, "script"="movej([3.1412,-1.5708,0,-1.5708,3.1412,5.8904], a=0.5, v=0.25, t=0, r=0)") -> ()  [unwired: 2 in, 4 out]
              }
            }
          }
        }
        n300 = case shown="True" "Move to particular posture" {
          tunnel: w48 -> [_ w464]
          frame False {
          }
          frame True {
            n301 = flat-sequence {
              tunnel: w464 -> [w466]
              frame #0 {
                n302 = invoke class="PrimaryInterfaceScript" method="Send"(reference=w466, "script"="movej([-1.5,-1.5,-2,-0.5,1.8,0], a=1.4, v=1.05, t=0, r=0)") -> ()  [unwired: 2 in, 4 out]
              }
            }
          }
        }
        n303 = property class="PrimaryInterfaceClientInternal"(reference=w40) -> ("RobotModeData"=w66:refnum<k24>)  [unwired: 1 in, 2 out]
        n304 = property class="PrimaryInterfaceClientInternal"(reference=w40) -> ("CartesianInfo"=w47:refnum<k24>)  [unwired: 1 in, 2 out]
        n305 = property class="RobotModeDataPackageEventArgs"(reference=w66) -> ("RobotPowerOn"=→"Powered on":bool)  [unwired: 1 in, 2 out]
        n306 = constructor class="SocketCommunicationServer"() -> (reference out=w59:refnum<k24>)  [unwired: 3 in, 2 out]
        n307 = property class="SocketCommunicationServer"(reference=w59) -> ("Enabled"=→"Enabled":bool)  [unwired: 1 in, 2 out]
        n308 = property class="SocketCommunicationServer"(reference=w59) -> ("Port"=→"Port":i32)  [unwired: 1 in, 2 out]
        n309 = property class="CartesianInfoPackageEventArgs"(reference=w47) -> ("TCPOffsetX"=→"TCPOffsetX":dbl)  [unwired: 1 in, 2 out]
        n310 = property class="CartesianInfoPackageEventArgs"(reference=w47) -> ("TCPOffsetY"=→"TCPOffsetY":dbl)  [unwired: 1 in, 2 out]
        n311 = property class="CartesianInfoPackageEventArgs"(reference=w47) -> ("TCPOffsetRX"=→"TCPOffsetRX":dbl)  [unwired: 1 in, 2 out]
        n312 = property class="CartesianInfoPackageEventArgs"(reference=w47) -> ("TCPOffsetRY"=→"TCPOffsetRY":dbl)  [unwired: 1 in, 2 out]
        n313 = property class="CartesianInfoPackageEventArgs"(reference=w47) -> ("Y"=→"Y":dbl)  [unwired: 1 in, 2 out]
        n314 = property class="CartesianInfoPackageEventArgs"(reference=w47) -> ("TCPOffsetZ"=→"TCPOffsetZ":dbl)  [unwired: 1 in, 2 out]
        n315 = property class="CartesianInfoPackageEventArgs"(reference=w47) -> ("TCPOffsetRZ"=→"TCPOffsetRZ":dbl)  [unwired: 1 in, 2 out]
        n316 = property class="CartesianInfoPackageEventArgs"(reference=w47) -> ("Ry"=→"Ry":dbl)  [unwired: 1 in, 2 out]
        n317 = property class="CartesianInfoPackageEventArgs"(reference=w47) -> ("Z"=→"Z":dbl)  [unwired: 1 in, 2 out]
        n318 = property class="CartesianInfoPackageEventArgs"(reference=w47) -> ("Rz"=→"Rz":dbl)  [unwired: 1 in, 2 out]
        n319 = property class="CartesianInfoPackageEventArgs"(reference=w47) -> ("X"=→"X":dbl)  [unwired: 1 in, 2 out]
        n320 = property class="CartesianInfoPackageEventArgs"(reference=w47) -> ("Rx"=→"Rx":dbl)  [unwired: 1 in, 2 out]
      }
    }
    n321 = property class="UR"(reference=w31) -> ("Dashboard"=w35:refnum<k24>)  [unwired: 1 in, 2 out]
    n322 = case shown="True" "Power off" {
      tunnel: w35 -> [_ w473]
      frame False {
      }
      frame True {
        n323 = flat-sequence {
          tunnel: w473 -> [w474]
          frame #0 {
            n324 = invoke class="DashboardClientInternal" method="PowerOff"(reference=w474) -> ()  [unwired: 2 in, 3 out]
          }
        }
      }
    }
    n325 = case shown="True" "Power on\nRelease brake" {
      tunnel: w35 -> [_ w475]
      frame False {
      }
      frame True {
        n326 = flat-sequence {
          tunnel: w475 -> [w477]
          frame #0 {
            n327 = invoke class="DashboardClientInternal" method="PowerOn"(reference=w477) -> (reference out=w476:refnum<k24>)  [unwired: 2 in, 2 out]
            n328 = invoke class="DashboardClientInternal" method="ReleaseBrake"(reference=w476) -> ()  [unwired: 2 in, 3 out]
          }
        }
      }
    }
  }
  n329 = invoke class="UR" method="RegisterLicense"(reference=w25, "licensee"="your company name", "key"="") -> (reference out=w27:refnum<k24>)  [unwired: 2 in, 4 out]
  n330 = control-ref of="Script to execute"() -> (w24:refnum<vi>)
  n331 = property class="Str"(reference=w24, "Value"="movej([-1.5,-1.5,-2,-0.5,1.8,0], a=1.4, v=1.05, t=0, r=0)") -> ()  [unwired: 1 in, 2 out]
  n332 = property class="UR"(reference=w27) -> ("LicenseInfo"=w26:refnum<k24>)  [unwired: 1 in, 2 out]
  n333 = invoke class="LicenseInfo" method="ToString"(reference=w26) -> ("ToString"=→"License state":string)  [unwired: 2 in, 2 out]
  n334 = while {
    stop <- "stop" stop-if-true
    n335 = global read "Global 1.vi" "TCP 스위치"() -> (w482:bool)
    n336 = case shown="True" w482 {
      frame False {
      }
      frame True {
        w504 = 4 ("length (rest)")
        n337 = global read "Global 1.vi" "몇번 병을 볼것인가"() -> (w494:string)
        n338 = TCP Open Connection(address="localhost", remote port or service name=u16 9999) -> (connection ID=w498:refnum<k5>, error out=w497:errorcluster)  [unwired: 3 in]
        n339 = TCP Write(connection ID=w498, data in=w494, error in (no error)=w497) -> (connection ID out=w496:refnum<k5>, error out=w495:errorcluster)  [unwired: 1 in, 1 out]
        n340 = TCP Read(connection ID=w496, error in (no error)=w495) -> (connection ID out=w513:refnum<k5>, data out=w487:string, error out=w512:errorcluster)  [unwired: 3 in]
        "지호씨가보낸 총좌표" <- w487
        n341 = String Subset(string=w487, offset (0)=8, length (rest)=w504) -> (substring=→"Z_havetogo":string)
        n342 = String Subset(string=w487, offset (0)=13, length (rest)=w504) -> (substring=→"RX_havetogo":string)
        n343 = String Subset(string=w487, offset (0)=4, length (rest)=w504) -> (substring=→"Y_havetogo":string)
        n344 = String Subset(string=w487, offset (0)=0, length (rest)=w504) -> (substring=→"X_havetogo":string)
        n345 = String Subset(string=w487, offset (0)=12, length (rest)=1 ("length (rest)")) -> (substring=→"Rx부호":string)
        n346 = String Subset(string=w487, offset (0)=23, length (rest)=w504) -> (substring=→"RZ_havetogo":string)
        n347 = String Subset(string=w487, offset (0)=18, length (rest)=w504) -> (substring=→"RY_havetogo":string)
        n348 = String Subset(string=w487, offset (0)=17, length (rest)=1 ("length (rest)")) -> (substring=→"Ry부호":string)
        n349 = String Subset(string=w487, offset (0)=22, length (rest)=1 ("length (rest)")) -> (substring=→"Rz부호":string)
        n350 = TCP Close Connection(connection ID=w513, error in (no error)=w512) -> ()  [unwired: 1 in, 2 out]
      }
    }
  }
